vi "Begin.vi"(8 "error in":errorcluster) -> (0 "error out":errorcluster)   [LabVIEW 2019]
doc: "Called before other user functions, this VI is expected to open initial I/O refnums, load in file data, and do all program initialization. Notice that the <B>error out</B> terminal is simply used for data flow. Wiring it to other structures or subVIs ensures that this VI runs first."
uses:
  <vilib>/Rock Robotics/WPI/DriverStation/WPI_DriverStationRobotMode2.ctl
  <vilib>/Rock Robotics/WPI/Joystick/WPI_JoystickDeviceEnum.ctl
  Subsystems/Turret/Turret_Cluster.ctl
  <vilib>/Rock Robotics/WPI/ThirdParty/Phoenix-LabVIEW/Motor Controller/Controls/CTRE_Phoenix_MotorControl_ControlMode.ctl
  Subsystems/Drive/DriveExecuteCluster.ctl
  Subsystems/Drive/DriveSetCluster.ctl
  <vilib>/Rock Robotics/WPI/ThirdParty/REV Robotics/SPARK MAX/Typedef/Spark MAX Motor Type.ctl
  Robot Global Data.vi
  Subsystems/Turret/Turret_Globals.vi
  Drive_Globals.vi
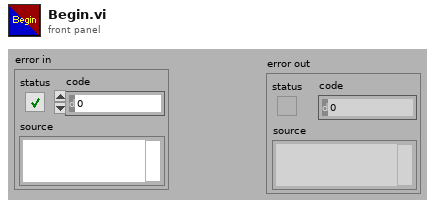
[diagram p1: front panel]
types:
  T1 = typedef "CTRE_Phoenix_MotorControl_ControlMode.ctl" = u16
  T2 = typedef "Spark MAX Motor Type.ctl" = enum16{"Brushed", "Brushless"}
  T3 = typedef "DriveSetCluster.ctl" = cluster{"Front/Back":dbl, "Turn":dbl, "Speed_Control?":bool}
  T4 = typedef "DriveExecuteCluster.ctl" = cluster{"Front/Back":dbl, "Turn":dbl, "Drive Control Type":enum16{"PercentVoltage", "SpeedControl"}}
  T5 = enum16{"FollowerType_PercentOutput", "FollowerType_AuxOutput1"}
  T6 = typedef "WPI_JoystickDeviceEnum.ctl" = enum16{"USB 0", "USB 1", "USB 2", "USB 3", "USB 4", "USB 5"}
  T7 = typedef "Turret_Cluster.ctl" = cluster{"Control_State":enum16{"Manual_PercentVoltage", "Manual_SpeedControl", "Auto_Targeting", "Position"}, "Spin_Power":dbl, "Flywheel_Power":dbl, "Going_To_Position":bool}
  T8 = typedef "WPI_DriverStationRobotMode2.ctl" = enum16{"Autonomous Disabled", "Autonomous Enabled", "Teleop Disabled", "Teleop Enabled", "Disconnected", "Finish", "Test Disabled", "Test Enabled", "Emergency Stopped"}
  T9 = typedef "WPI_MotorControlDeviceRef.ctl" = cluster{"DeviceStatus":errorcluster, "Type":T10, "PWM":cluster{"PWM Channel":T11, "DeadBand":T12}, "CAN":cluster{"Device Number":u8, "SetOutput VI Ref":variant, "GetOutput VI Ref":variant, "Enable VI Ref":variant, "Disable VI Ref":variant, "Data":variant}, "Invert":bool, "DIO PWM":cluster{"PWM \"Enable\" Channel":T11, "DIOChannel":T13, "PWM Rate":dbl}}
  T10 = typedef "WPI_MotorControlType.ctl" = enum16{"PWM", "CAN", "DIO PWM"}
  T11 = typedef "FPGA_DIOPWMChannel.ctl" = enum8{"PWM 0", "PWM 1", "PWM 2", "PWM 3", "PWM 4", "PWM 5", "PWM 6", "PWM 7", "PWM 8", "PWM 9", "PWM MXP 0", "PWM MXP 1", "PWM MXP 2", "PWM MXP 3", "PWM MXP 4", "PWM MXP 5", "PWM MXP 6", "PWM MXP 7", "PWM MXP 8", "PWM MXP 9", "Invalid"}
  T12 = typedef "WPI_PWMDeadband.ctl" = cluster{"Name":string, "maxPositivePwm":i32, "minPositivePwm":i32, "centerPwm":i32, "maxNegativePwm":i32, "minNegativePwm":i32, "angularRange":u16}
  T13 = typedef "FPGA_DIOChannel.ctl" = enum8{"DIO 0", "DIO 1", "DIO 2", "DIO 3", "DIO 4", "DIO 5", "DIO 6", "DIO 7", "DIO 8", "DIO 9", "DIO MXP 0", "DIO MXP 1", "DIO MXP 2", "DIO MXP 3", "DIO MXP 4", "DIO MXP 5", "DIO MXP 6", "DIO MXP 7", "DIO MXP 8", "DIO MXP 9", "DIO MXP 10", "DIO MXP 11", "DIO MXP 12", "DIO MXP 13", "DIO MXP 14", "DIO MXP 15", "SPI Port CS1", "SPI Port CS2", "SPI Port CS3", "SPI Port MISO", "SPI Port MOSI", "Invalid"}
  T14 = typedef "WPI_JoystickDevRef.ctl" = cluster{"Device":T6}
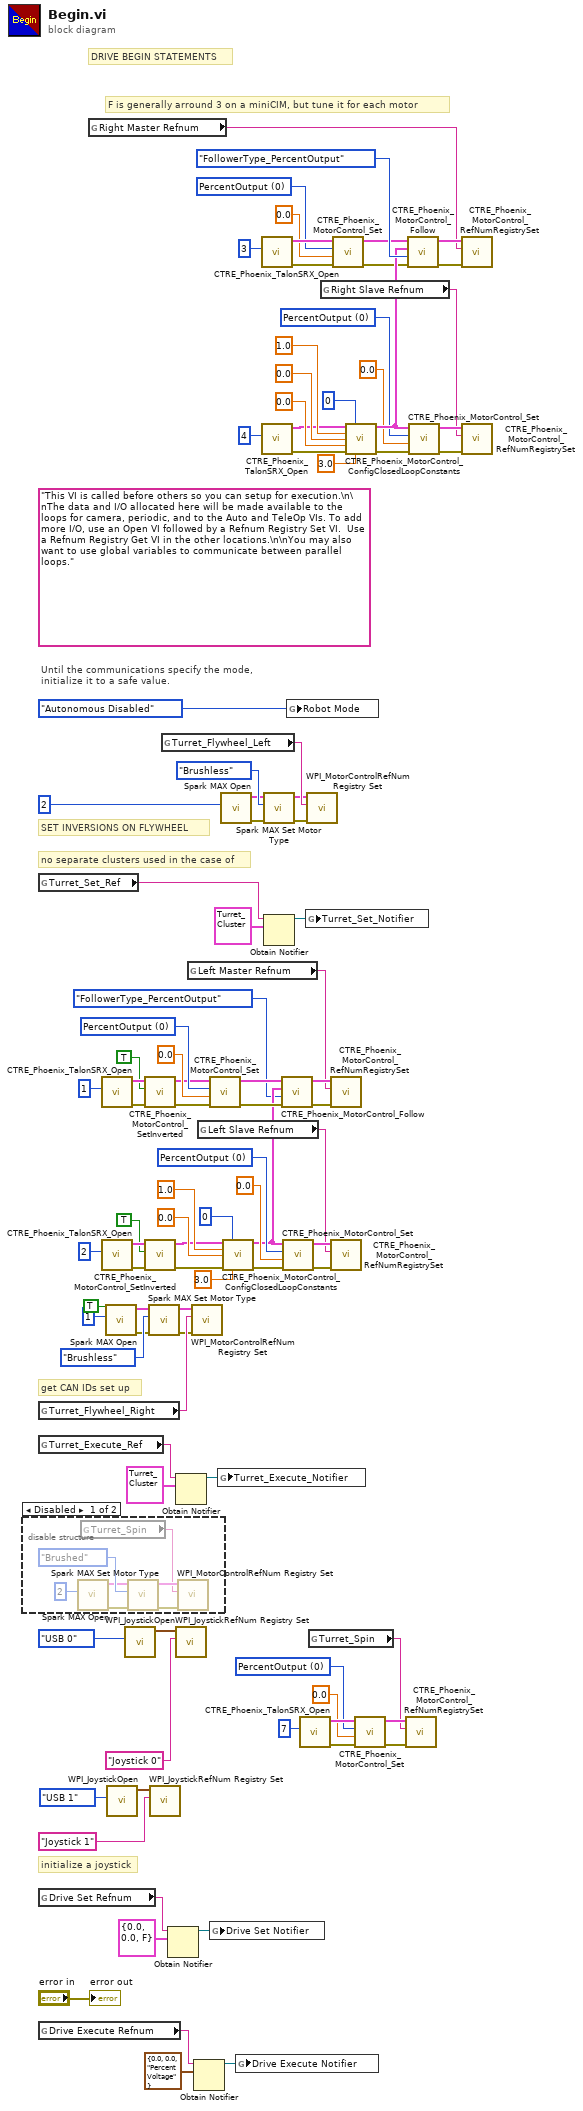
[diagram p0: block diagram]
diagram:
  w8 = T1 0 items=["PercentOutput"=0, "Position"=1, "Velocity"=2, "Current"=3, "Follower"=5, "MotionProfile"=6, "MotionMagic"=7, "MotionProfileArc"=10, "Disabled"=15] ("Control Mode")
  w52 = T1 0 items=["PercentOutput"=0, "Position"=1, "Velocity"=2, "Current"=3, "Follower"=5, "MotionProfile"=6, "MotionMagic"=7, "MotionProfileArc"=10, "Disabled"=15] ("Control Mode")
  w47 = T1 0 items=["PercentOutput"=0, "Position"=1, "Velocity"=2, "Current"=3, "Follower"=5, "MotionProfile"=6, "MotionMagic"=7, "MotionProfileArc"=10, "Disabled"=15] ("Control Mode")
  w82 = T1 0 items=["PercentOutput"=0, "Position"=1, "Velocity"=2, "Current"=3, "Follower"=5, "MotionProfile"=6, "MotionMagic"=7, "MotionProfileArc"=10, "Disabled"=15] ("Control Mode")
  w85 = T1 0 items=["PercentOutput"=0, "Position"=1, "Velocity"=2, "Current"=3, "Follower"=5, "MotionProfile"=6, "MotionMagic"=7, "MotionProfileArc"=10, "Disabled"=15] ("Control Mode")
  (unwired) "This VI is called before others so you can setup for execution.\n\nThe data and I/O allocated here will be made available to the loops for camera, periodic, and to the Auto and TeleOp VIs. To add more I/O, use an Open VI followed by a Refnum Registry Set VI.  Use a Refnum Registry Get VI in the other locations.\n\nYou may also want to use global variables to communicate between parallel loops."
  # "get CAN IDs set up"
  # "no separate clusters used in the case of"
  # "DRIVE BEGIN STATEMENTS"
  # "F is generally arround 3 on a miniCIM, but tune it for each motor"
  # "SET INVERSIONS ON FLYWHEEL"
  # "initialize a joystick"
  # "Until the communications specify the mode,\ninitialize it to a safe value."
  n1 = disable-structure shown="Disabled" {
    frame Disabled {
      n2 = call <vilib>:"Spark MAX Open.vi"("Device Number"=u8 2) -> ("error out"=w104:errorcluster, "MotorControlDeviceRef"=w105:T9)  [unwired: 9 in]
      n3 = global read "Turret_Globals.vi" "Turret_Spin"() -> (w101:string)
      n4 = call <vilib>:"Spark MAX Set Motor Type.vi"("error in (no error)"=w104, "Motor Type"=Spark_MAX_Motor_Type."Brushed", "MotorControlDevRef"=w105) -> ("error out"=w102:errorcluster, "MotorControlDeviceRef"=w103:T9)  [unwired: 7 in]
      n5 = call <vilib>:"WPI_MotorControlRefNum Registry Set.vi"("error in (no error)"=w102, "refnum name"=w101, "MotorControlDevRef"=w103) -> ()  [unwired: 7 in, 2 out]
    }
    frame Enabled {
    }
  }
  n6 = global read "Turret_Globals.vi" "Turret_Set_Ref"() -> (w93:string)
  n7 = global read "Turret_Globals.vi" "Turret_Flywheel_Right"() -> (w12:string)
  n8 = global read "Turret_Globals.vi" "Turret_Execute_Ref"() -> (w92:string)
  n9 = global read "Drive_Globals.vi" "Drive Set Refnum"() -> (w38:string)
  n10 = global read "Drive_Globals.vi" "Drive Execute Refnum"() -> (w37:string)
  n11 = global read "Drive_Globals.vi" "Right Master Refnum"() -> (w44:string)
  n12 = call <vilib>:"CTRE_Phoenix_TalonSRX_Open.vi"("Device Number"=u8 1) -> ("error out"=w33:errorcluster, "CAN Talon SRX Ref"=w32:T9)  [unwired: 9 in]
  n13 = call <vilib>:"CTRE_Phoenix_TalonSRX_Open.vi"("Device Number"=u8 2) -> ("error out"=w28:errorcluster, "CAN Talon SRX Ref"=w29:T9)  [unwired: 9 in]
  n14 = call <vilib>:"Spark MAX Open.vi"("Invert"=TRUE, "Device Number"=u8 1) -> ("error out"=w2:errorcluster, "MotorControlDeviceRef"=w15:T9)  [unwired: 8 in]
  n15 = call <vilib>:"WPI_JoystickOpen.vi"("JoystickDevice"=WPI_JoystickDeviceEnum."USB 1") -> ("JoystickDevRef"=w88:T14)  [unwired: 10 in]
  n16 = call <vilib>:"WPI_JoystickOpen.vi"("JoystickDevice"=WPI_JoystickDeviceEnum."USB 0") -> ("JoystickDevRef"=w98:T14)  [unwired: 10 in]
  n17 = call <vilib>:"CTRE_Phoenix_MotorControl_SetInverted.vi"("error in (no error)"=w33, "Invert?"=TRUE, "PhoenixMotorControlDevRef"=w32) -> ("error out"=w30:errorcluster, "PhoenixMotorControlDevRef"=w31:T9)  [unwired: 7 in]
  n18 = call <vilib>:"CTRE_Phoenix_MotorControl_SetInverted.vi"("error in (no error)"=w28, "Invert?"=TRUE, "PhoenixMotorControlDevRef"=w29) -> ("error out"=w27:errorcluster, "PhoenixMotorControlDevRef"=w26:T9)  [unwired: 7 in]
  n19 = call <vilib>:"Spark MAX Set Motor Type.vi"("error in (no error)"=w2, "Motor Type"=Spark_MAX_Motor_Type."Brushless", "MotorControlDevRef"=w15) -> ("error out"=w1:errorcluster, "MotorControlDeviceRef"=w16:T9)  [unwired: 7 in]
  n20 = call <vilib>:"WPI_JoystickRefNum Registry Set.vi"("refnum name"="Joystick 1", "JoystickDevRef"=w88) -> ()  [unwired: 8 in, 2 out]
  n21 = global read "Turret_Globals.vi" "Turret_Flywheel_Left"() -> (w23:string)
  n22 = Obtain Notifier(name (unnamed)=w38, notification data type=T3 {"Front/Back"=0.0, "Turn"=0.0, "Speed_Control?"=FALSE} ("Drive Set Cluster")) -> (notifier out=w34:refnum<notifier>)  [unwired: 2 in, 2 out]
  n23 = Obtain Notifier(name (unnamed)=w92, notification data type=T7 {"Control_State"=enum."Manual_PercentVoltage", "Spin_Power"=0.0, "Flywheel_Power"=0.0, "Going_To_Position"=FALSE}) -> (notifier out=w90:refnum<notifier>)  [unwired: 2 in, 2 out]
  n24 = call <vilib>:"WPI_JoystickRefNum Registry Set.vi"("refnum name"="Joystick 0", "JoystickDevRef"=w98) -> ()  [unwired: 8 in, 2 out]
  n25 = global read "Drive_Globals.vi" "Left Master Refnum"() -> (w42:string)
  n26 = call <vilib>:"WPI_MotorControlRefNum Registry Set.vi"("error in (no error)"=w1, "refnum name"=w12, "MotorControlDevRef"=w16) -> ()  [unwired: 7 in, 2 out]
  n27 = Obtain Notifier(name (unnamed)=w37, notification data type=T4 {"Front/Back"=0.0, "Turn"=0.0, "Drive Control Type"=enum."PercentVoltage"}) -> (notifier out=w36:refnum<notifier>)  [unwired: 2 in, 2 out]
  n28 = global read "Drive_Globals.vi" "Left Slave Refnum"() -> (w45:string)
  n29 = call <vilib>:"CTRE_Phoenix_MotorControl_Set.vi"("error in (no error)"=w30, "Output"=0.0, "Control Mode"=w85, "PhoenixMotorControlDevRef"=w31) -> ("error out"=w74:errorcluster, "PhoenixMotorControlDevRef"=w73:T9)  [unwired: 6 in]
  n30 = global write "Drive_Globals.vi" "Drive Set Notifier"(w34) -> ()
  n31 = global write "Turret_Globals.vi" "Turret_Execute_Notifier"(w90) -> ()
  n32 = call <vilib>:"Spark MAX Open.vi"("Device Number"=u8 2) -> ("error out"=w20:errorcluster, "MotorControlDeviceRef"=w19:T9)  [unwired: 9 in]
  n33 = call <vilib>:"CTRE_Phoenix_MotorControl_ConfigClosedLoopConstants.vi"("PhoenixMotorControlDevRef"=w26, "slotIdx"=0, "P"=1.0, "I"=0.0, "error in (no error)"=w27, "F"=3.0) -> ("PhoenixMotorControlDevRef"=w70:T9, "error out"=w78:errorcluster)  [unwired: 8 in]
  n34 = global write "Drive_Globals.vi" "Drive Execute Notifier"(w36) -> ()
  n35 = call <vilib>:"CTRE_Phoenix_TalonSRX_Open.vi"("Device Number"=u8 3) -> ("error out"=w50:errorcluster, "CAN Talon SRX Ref"=w49:T9)  [unwired: 9 in]
  n36 = call <vilib>:"CTRE_Phoenix_TalonSRX_Open.vi"("Device Number"=u8 4) -> ("error out"=w57:errorcluster, "CAN Talon SRX Ref"=w56:T9)  [unwired: 9 in]
  n37 = call <vilib>:"Spark MAX Set Motor Type.vi"("error in (no error)"=w20, "Motor Type"=Spark_MAX_Motor_Type."Brushless", "MotorControlDevRef"=w19) -> ("error out"=w18:errorcluster, "MotorControlDeviceRef"=w17:T9)  [unwired: 7 in]
  n38 = Obtain Notifier(name (unnamed)=w93, notification data type=T7 {"Control_State"=enum."Manual_PercentVoltage", "Spin_Power"=0.0, "Flywheel_Power"=0.0, "Going_To_Position"=FALSE}) -> (notifier out=w91:refnum<notifier>)  [unwired: 2 in, 2 out]
  n39 = call <vilib>:"CTRE_Phoenix_MotorControl_Follow.vi"("error in (no error)"=w74, "FollowerType"=T5."FollowerType_PercentOutput", "Master Controller to Follow"=w70, "PhoenixMotorControlDevRef"=w73) -> ("error out"=w71:errorcluster, "PhoenixMotorControlDevRef"=w72:T9)  [unwired: 6 in]
  n40 = call <vilib>:"CTRE_Phoenix_MotorControl_Set.vi"("error in (no error)"=w78, "Output"=0.0, "Control Mode"=w82, "PhoenixMotorControlDevRef"=w70) -> ("error out"=w80:errorcluster, "PhoenixMotorControlDevRef"=w81:T9)  [unwired: 6 in]
  n41 = global write "Robot Global Data.vi" "Robot Mode"(WPI_DriverStationRobotMode2."Autonomous Disabled" ("Robot Mode")) -> ()
  n42 = call <vilib>:"CTRE_Phoenix_TalonSRX_Open.vi"("Device Number"=u8 7) -> ("error out"=w11:errorcluster, "CAN Talon SRX Ref"=w10:T9)  [unwired: 9 in]
  n43 = global write "Turret_Globals.vi" "Turret_Set_Notifier"(w91) -> ()
  n44 = call <vilib>:"WPI_MotorControlRefNum Registry Set.vi"("error in (no error)"=w18, "refnum name"=w23, "MotorControlDevRef"=w17) -> ()  [unwired: 7 in, 2 out]
  n45 = global read "Turret_Globals.vi" "Turret_Spin"() -> (w5:string)
  n46 = global read "Drive_Globals.vi" "Right Slave Refnum"() -> (w43:string)
  n47 = call <vilib>:"CTRE_Phoenix_MotorControl_RefNumRegistrySet.vi"("error in (no error)"=w71, "refnum name"=w42, "PhoenixMotorControlDevRef"=w72) -> ()  [unwired: 7 in, 2 out]
  n48 = call <vilib>:"CTRE_Phoenix_MotorControl_RefNumRegistrySet.vi"("error in (no error)"=w80, "refnum name"=w45, "PhoenixMotorControlDevRef"=w81) -> ()  [unwired: 7 in, 2 out]
  n49 = call <vilib>:"CTRE_Phoenix_MotorControl_Set.vi"("error in (no error)"=w50, "Output"=0.0, "Control Mode"=w47, "PhoenixMotorControlDevRef"=w49) -> ("error out"=w63:errorcluster, "PhoenixMotorControlDevRef"=w64:T9)  [unwired: 6 in]
  n50 = call <vilib>:"CTRE_Phoenix_MotorControl_ConfigClosedLoopConstants.vi"("PhoenixMotorControlDevRef"=w56, "slotIdx"=0, "P"=1.0, "I"=0.0, "D"=0.0, "error in (no error)"=w57, "F"=3.0) -> ("PhoenixMotorControlDevRef"=w67:T9, "error out"=w58:errorcluster)  [unwired: 7 in]
  n51 = call <vilib>:"CTRE_Phoenix_MotorControl_Set.vi"("error in (no error)"=w11, "Output"=0.0, "Control Mode"=w8, "PhoenixMotorControlDevRef"=w10) -> ("error out"=w7:errorcluster, "PhoenixMotorControlDevRef"=w6:T9)  [unwired: 6 in]
  n52 = call <vilib>:"CTRE_Phoenix_MotorControl_RefNumRegistrySet.vi"("error in (no error)"=w7, "refnum name"=w5, "PhoenixMotorControlDevRef"=w6) -> ()  [unwired: 7 in, 2 out]
  n53 = call <vilib>:"CTRE_Phoenix_MotorControl_Follow.vi"("error in (no error)"=w63, "FollowerType"=T5."FollowerType_PercentOutput", "Master Controller to Follow"=w67, "PhoenixMotorControlDevRef"=w64) -> ("error out"=w66:errorcluster, "PhoenixMotorControlDevRef"=w65:T9)  [unwired: 6 in]
  n54 = call <vilib>:"CTRE_Phoenix_MotorControl_Set.vi"("error in (no error)"=w58, "Output"=0.0, "Control Mode"=w52, "PhoenixMotorControlDevRef"=w67) -> ("error out"=w54:errorcluster, "PhoenixMotorControlDevRef"=w53:T9)  [unwired: 6 in]
  n55 = call <vilib>:"CTRE_Phoenix_MotorControl_RefNumRegistrySet.vi"("error in (no error)"=w66, "refnum name"=w44, "PhoenixMotorControlDevRef"=w65) -> ()  [unwired: 7 in, 2 out]
  n56 = call <vilib>:"CTRE_Phoenix_MotorControl_RefNumRegistrySet.vi"("error in (no error)"=w54, "refnum name"=w43, "PhoenixMotorControlDevRef"=w53) -> ()  [unwired: 7 in, 2 out]
  "error out" <- "error in"
